vi "Control_PID_proiect.vi"() -> ()   [LabVIEW 2025]
uses:
  <vilib>/addons/control/pid/pid.llb/PID (DBL).vi
  <vilib>/addons/control/pid/NI_PID_pid.lvlib
  <vilib>/measure/NI_MABase.lvlib
panel:
  out "Waveform Graph":waveform(dbl)(graph)
  out "?":dbl
  out "Perioada":dbl
  out "MAX_PID)":dbl
  out "Eroarea stationara":dbl
  in  "amplitude":dbl(knob)=1.0 scale=0.0..10.0
  in  "frequency":dbl(knob)=10.0 scale=0.0..10.0
  out "Waveform Chart":cluster{"setpoint":dbl, dbl}(graph)
  in  "stop":bool
  in  "PID gains":T1={"proportional gain (Kc)"=1.0, "integral time (Ti, min)"=0.01, "derivative time (Td, min)"=0.0} {"derivative time (Td, min)" format="%.3f"; "integral time (Ti, min)" format="%.3f"; "proportional gain (Kc)" format="%.3f"}
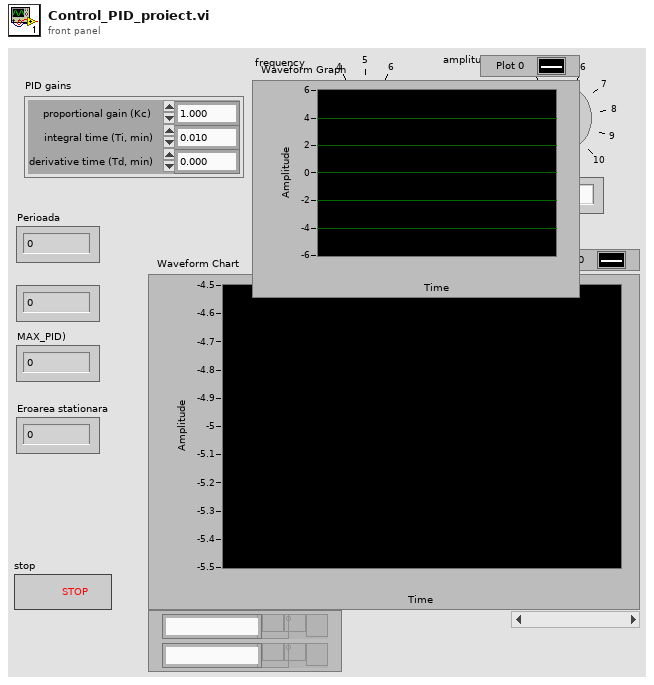
[diagram p1: front panel]
types:
  T1 = cluster{"proportional gain (Kc)":dbl, "integral time (Ti, min)":dbl, "derivative time (Td, min)":dbl}
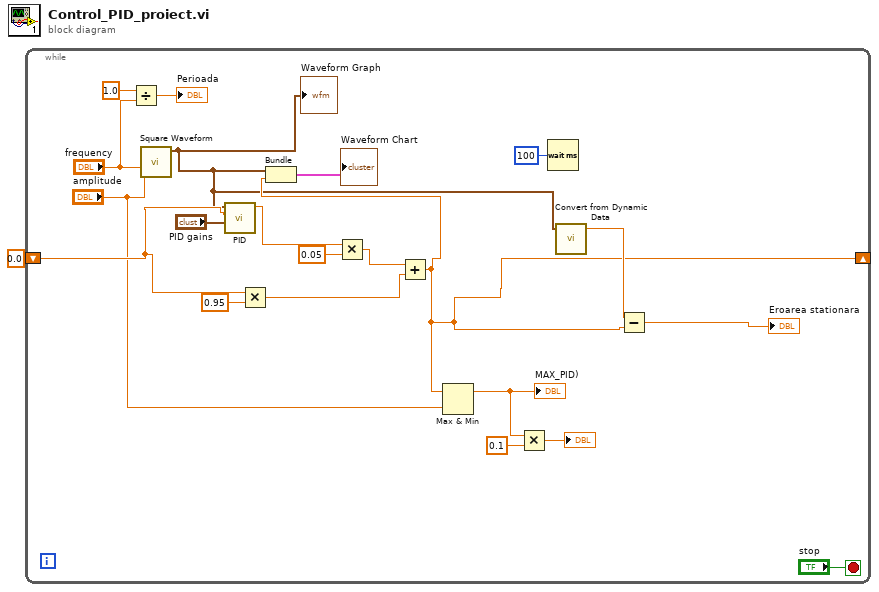
[diagram p0: block diagram]
diagram:
  n1 = while {
    shift-right: [w10] -> _
    shift-left: 0.0 -> [w13]
    stop <- "stop" stop-if-true
    n2 = Divide(x=1.0, y="frequency") -> (x/y=→"Perioada":dbl)
    n3 = call <vilib>:"Square Waveform.vi"("amplitude"="amplitude", "frequency"="frequency") -> ("signal out"=w2:waveform(dbl))  [unwired: 8 in, 1 out]
    "Waveform Graph" <- w2
    n4 = call-poly <vilib>:"PID.vi"("PID gains"="PID gains", "process variable"=w13, "setpoint"=w2) -> ("output"=w19:dbl)  [unwired: 7 in, 1 out]
    n5 = Multiply(x=w13, y=0.95) -> (x*y=w16:dbl)
    n6 = Multiply(x=w19, y=0.05) -> (x*y=w17:dbl)
    n7 = Add(x=w17, y=w16) -> (x+y=w10:dbl)
    n8 = Bundle "Bundle"("signal out"=w2, w10) -> (→"Waveform Chart":cluster{"signal out":waveform(dbl), dbl})  [unwired: 1 in]
    n9 = Max & Min(x=w10, y="amplitude") -> (max(x,y)=w5:dbl)  [unwired: 1 out]
    "MAX_PID)" <- w5
    n10 = Multiply(x=w5, y=0.1) -> (x*y=→"?":dbl)
    n11 = Wait (ms)(milliseconds to wait=u32 100) -> ()  [unwired: 1 out]
    n12 = call "Convert from Dynamic Data"("Dynamic Data Type"=w2) -> ("Scalar"=w12:dbl)  [unwired: 3 in]
    n13 = Subtract(x=w12, y=w10) -> (x-y=→"Eroarea stationara":dbl)
  }
